vi "M3102A channel daq config.vi"(5 "DAQ":T1={"cycles"=1, "points"=100, "triggerMode"=0, "triggerDelay"=0} {"triggerMode" items=["Auto", "VI/HVI", "External", "Analog"]; "cycles" min=0}, 6 "nChannel":i32, 7 "Channel":T2={"fullscale"=0.5, "impedance"=1, "coupling"=0} {"coupling" items=["DC", "AC"]; "impedance" items=["High Z", "50 Ohms"]; "fullscale" items=["0.0625"=0.0625, "0.125"=0.125, "0.25"=0.25, "0.5"=0.5, "1"=1.0, "2"=2.0, "4"=4.0]}, 8 "errorIn":errorcluster, 11 "moduleID":i32) -> (0 "errorOut":errorcluster, 3 "moduleIDout":i32)   [LabVIEW 2021]
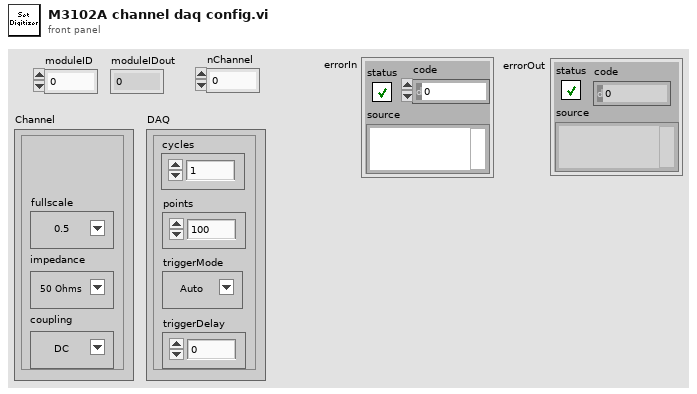
[diagram p1: front panel]
types:
  T1 = cluster{"cycles":i32, "points":i32, "triggerMode":i32, "triggerDelay":i32}
  T2 = cluster{"fullscale":dbl, "impedance":i32, "coupling":i32}
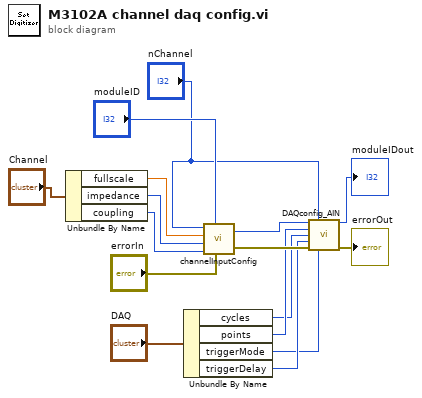
[diagram p0: block diagram]
diagram:
  n1 = Unbundle By Name("Channel") -> ("fullscale"=w9:dbl, "impedance"=w8:i32, "coupling"=w7:i32)
  n2 = Unbundle By Name("DAQ") -> ("cycles"=w4:i32, "points"=w5:i32, "triggerMode"=w2:i32, "triggerDelay"=w3:i32)
  n3 = call <vilib>:"channelInputConfig.vi"("errorIn"="errorIn", "moduleID"="moduleID", "coupling"=w7, "impedance"=w8, "fullscale"=w9, "nChannel"="nChannel") -> ("errorOut"=w15:errorcluster, "moduleIDout"=w16:i32)
  n4 = call <vilib>:"DAQconfig_AIN.vi"("moduleID"=w16, "nDAQ"="nChannel", "DAQpointsPerCycle"=w5, "cycles"=w4, "triggerDelay"=w3, "errorIn"=w15, "triggerMode"=w2) -> ("moduleIDout"=→"moduleIDout":i32, "errorOut"=→"errorOut":errorcluster)  [unwired: 7 in]
